vi "Get Number of Records Done.vi"(8 "error in":errorcluster, 11 "FPGA VI Reference In":refnum<k20>) -> (0 "error out":errorcluster, 2 "Records Done":u32, 3 "FPGA VI Reference Out":refnum<k20>)   [LabVIEW 2012]
uses:
  <vilib>/Utility/error.llb/Error Cluster From Error Code.vi
  <vilib>/rvi/errors/niLvFpgaAdjustHostInterfaceError.vi
  <vilib>/rvi/interface/nirviReadWriteControl/nirviReadWriteControl.xnode
  NiFpgaLv.dll
  <vilib>/rvi/interface/Simulation/niFpgaSimulationCallBeginRW.vi
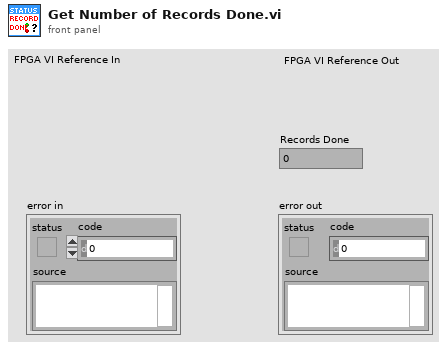
[diagram p1: front panel]
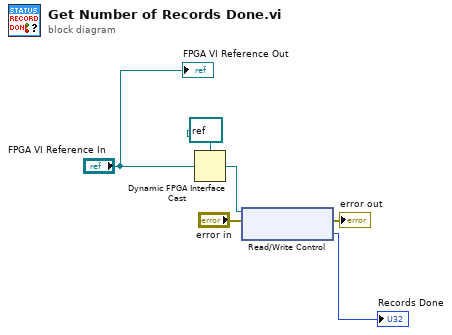
[diagram p0: block diagram]
diagram:
  n1 = Dynamic FPGA Interface Cast(Session In=refnum<k20> refnum ("Type"), Type="FPGA VI Reference In") -> (Session Out=w4:refnum<k20>)
  n2 = xnode "Read/Write Control"("FPGA VI Reference In"=w4, "error in"="error in") -> ("error out"=→"error out":errorcluster, "Records Done"=→"Records Done":u32)  [unwired: 1 out]
  "FPGA VI Reference Out" <- "FPGA VI Reference In"
